vi "Find Mutex.vi"(2 "Mutex Name":string, 3 "Mutex Collection":T1) -> (0 "Index":i32, 1 "Found?":bool)   [LabVIEW 2021]
uses:
  <vilib>/myRIO/Common/Instrument Driver Framework/Utilities/typedefs/Mutex Collection.ctl
  <vilib>/myRIO/Common/Instrument Driver Framework/Utilities/typedefs/Named Mutex.ctl
  <vilib>/myRIO/Common/Instrument Driver Framework/Utilities/typedefs/Reentrant Mutex.ctl
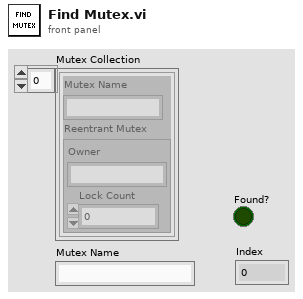
[diagram p1: front panel]
types:
  T1 = typedef "Mutex Collection.ctl" = T2[]
  T2 = typedef "Named Mutex.ctl" = cluster{"Mutex Name":string, "Reentrant Mutex":T3}
  T3 = typedef "Reentrant Mutex.ctl" = cluster{"Owner":string, "Lock Count":u32}
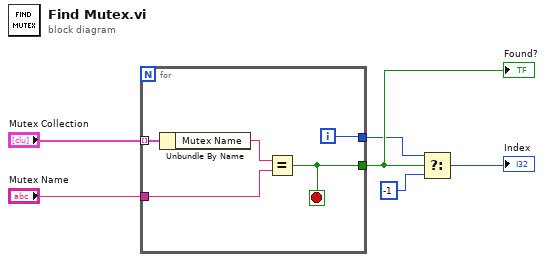
[diagram p0: block diagram]
diagram:
  n1 = for {
    tunnel: "Mutex Collection" -> [w11] mode=indexing
    tunnel: "Mutex Name" -> [w9]
    tunnel: [w8] -> w3
    tunnel: [w7] -> w4
    i -> [w8]
    stop <- w7 stop-if-true
    n2 = Unbundle By Name(w11) -> ("Mutex Name"=w10:string)
    n3 = Equal?(x=w10, y=w9) -> (x = y?=w7:bool)
  }
  "Found?" <- w4
  n4 = Select(t=w3, s=w4, f=-1) -> (s? t:f=→"Index":i32)
